vi "Get_Title.vi"() -> ()   [LabVIEW 2013]
panel:
  out "Title":string
  # "Use the Web Service Request input terminal to call the VIs on the Web Services palette. Do not remove it from the connector pane unless you don't need access to the palette."
  # "Each additional control wired to the connector pane will be available as an input in the URL. To include an indicator in terminal-mode output (the default setting), it must also be wired to the connector pane."
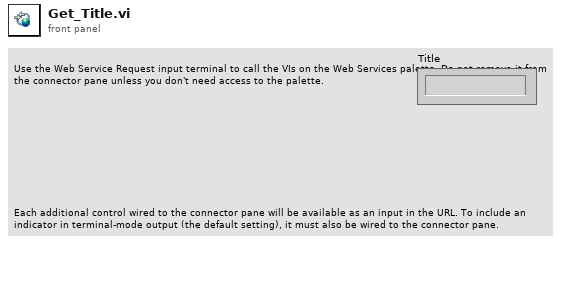
[diagram p1: front panel]
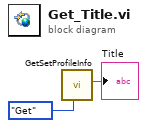
[diagram p0: block diagram]
diagram:
  n1 = call "GetSetProfileInfo.vi"("Get/Set State"=enum16{"Get", "Set", "Load"}."Get") -> ("Title"=→"Title":string)  [unwired: 8 in, 2 out]
